vi "Gyro.vi"   [LabVIEW 2014]
uses:
  Begin/Global RefNums.vi
  Begin/Global Variables.vi
  _Dependencies/NavX/navX-MXP IMU.lvlib
types:
  T1 = typedef "navX-MXP IMU.lvlib/navX Device TypeDef.ctl" = cluster{"navX Interface Protocol":T2, "navX Interface Protocol TypeDefs":cluster{"SPIDevRef":T3, "I2CDevRef":T6}, "navX System Information":cluster{"Board Information":T8, "Status":T9, "Offsets":T13}, "navX Common Information":cluster{"Update Rate (4Hz-60Hz)":T14, "refnum name":string, "error":errorcluster}}
  T2 = typedef "navX-MXP IMU.lvlib/navX Interface Protocol.ctl" = enum16{"SPI", "I2C"}
  T3 = typedef "WPI_SPIDevRef.ctl" = cluster{"DevStatus":errorcluster, "Handle":i32, "Controller":T4, "SPI Bus":T5}
  T4 = typedef "FPGA_TypedefDigitalModule.ctl" = enum16{"Controller 1"}
  T5 = typedef "spi_bus.ctl" = enum16{"SPI On-Board, CS0", "SPI On-Board, CS1", "SPI On-Board, CS2", "SPI On-Board, CS3", "SPI MXP", "Invalid"}
  T6 = typedef "WPI_I2CDevRef.ctl" = cluster{"DevStatus":errorcluster, "Controller":T4, "Device Address":u8, "Handle":i32, "I2C Bus":T7}
  T7 = typedef "i2c_bus.ctl" = enum16{"I2C On-Board", "I2C MXP", "Invalid"}
  T8 = typedef "navX-MXP IMU.lvlib/navX Board Information.ctl" = cluster{"WhoAmI (50 | 0x32)":u8, "Board Revision":u8, "Firmware Major Version":u8, "Firmware Minor Version":u8}
  T9 = typedef "navX-MXP IMU.lvlib/navX Status Data.ctl" = cluster{"Update Rate Hz":u8, "Accelerometer Full-Scale Range":u8, "Gyro Full-Scale Range":u16, "NAVX_OP_STATUS":T10, "NAVX_CAL_STATUS":T11, "NAVX_SELFTEST_STATUS":u8, "NAVX_SENSOR_STATUS":T12}
  T10 = typedef "navX-MXP IMU.lvlib/navX NAVX_OP_STATUS.ctl" = u8
  T11 = typedef "navX-MXP IMU.lvlib/navX NAVX_CAL_STATUS.ctl" = u8
  T12 = typedef "navX-MXP IMU.lvlib/navX NAVX_SENSOR_STATUS.ctl" = cluster{"MOVING":bool, "YAW_STABLE":bool, "MAG_DISTURBANCE":bool, "ALTITUDE_VALID":bool, "SEALEVEL_PRESS_SET":bool, "FUSED_HEADING_VALID":bool}
  T13 = typedef "navX-MXP IMU.lvlib/navX Offsets Data.ctl" = cluster{"Yaw":dbl, "Quat W":dbl, "Quat X":dbl, "Quat Y":dbl, "Quat Z":dbl}
  T14 = typedef "navX-MXP IMU.lvlib/navX Update Rate.ctl" = u8
  T15 = typedef "navX-MXP IMU.lvlib/navX YPRH Data.ctl" = cluster{"Yaw":dbl, "Pitch":dbl, "Roll":dbl, "Heading":dbl}
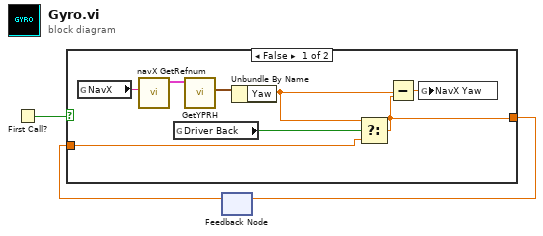
[diagram p0: block diagram]
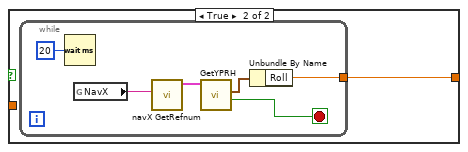
[diagram p2: hidden frame]
diagram:
  n1 = First Call?() -> (First Call?: T/F=w1:bool)
  n2 = feedback #1() -> (w3:dbl)  [unwired: 1 in]
  n3 = case shown="False" w1 {
    tunnel: [w7 w12] -> w2
    tunnel: w3 -> [w8 _]
    frame False {
      n4 = global read "Global RefNums.vi" "NavX"() -> (w9:string)
      n5 = call "navX GetRefnum.vi"("refnum name"=w9) -> ("navX Device TypeDef"=w5:T1)  [unwired: 9 in, 1 out]
      n6 = global read "Global Variables.vi" "Driver Back"() -> (w10:bool)
      n7 = call "GetYPRH.vi"("navX Device TypeDef"=w5) -> ("YPRH"=w6:T15)  [unwired: 8 in, 2 out]
      n8 = Unbundle By Name(w6) -> ("Yaw"=w4:dbl)
      n9 = Select(t=w4, s=w10, f=w8) -> (s? t:f=w7:dbl)
      n10 = Subtract(x=w4, y=w7) -> (x-y=w11:dbl)
      n11 = global write "Global Variables.vi" "NavX Yaw"(w11) -> ()
    }
    frame True {
      n12 = while {
        tunnel: [w13] -> w12
        stop <- w16 stop-if-true
        n13 = Wait (ms)(milliseconds to wait=u32 20) -> ()  [unwired: 1 out]
        n14 = global read "Global RefNums.vi" "NavX"() -> (w17:string)
        n15 = call "navX GetRefnum.vi"("refnum name"=w17) -> ("navX Device TypeDef"=w18:T1)  [unwired: 9 in, 1 out]
        n16 = call "GetYPRH.vi"("navX Device TypeDef"=w18) -> ("Valid?"=w16:bool, "YPRH"=w14:T15)  [unwired: 8 in, 1 out]
        n17 = Unbundle By Name(w14) -> ("Roll"=w13:dbl)
      }
    }
  }
  n18 = feedback-in #1(w2) -> ()
